vi "DUAL GAUGE-convert2int.vi"(0 "String in":string, 2 "W/R [W: Int in; Str out ]":bool, 9 "Integer1 in":u8, 11 "Integer2 in":u8) -> (4 "String out":string, 6 "Integer1 out":u8, 8 "Integer2 out":u8, 10 "Integer3 out":u8, 15 "Integer4 out":u8)   [LabVIEW 2010, in "Dual Gauge.lvlib"]
uses:
  Dual Gauge.lvlib
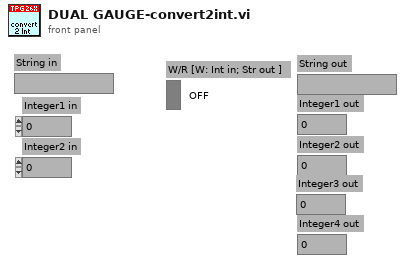
[diagram p1: front panel]
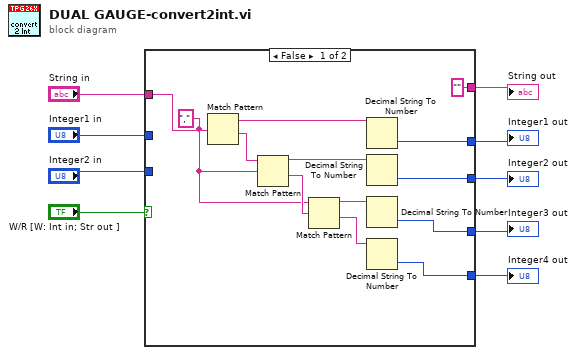
[diagram p0: block diagram]
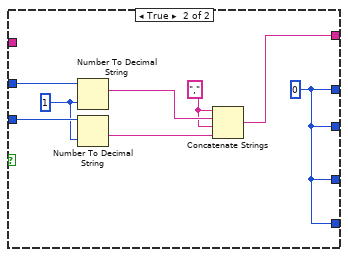
[diagram p2: hidden frame]
diagram:
  n1 = case shown="False" "W/R [W: Int in; Str out ]" {
    tunnel: "Integer1 in" -> [_ w30]
    tunnel: "Integer2 in" -> [_ w29]
    tunnel: ["" w28] -> w6
    tunnel: "String in" -> [w22 _]
    tunnel: [w20 w23] -> w4
    tunnel: [w19 w23] -> w3
    tunnel: [w12 w23] -> w2
    tunnel: [w11 w23] -> w1
    frame False {
      w10 = "," ("regular expression")
      n2 = Match Pattern(string=w22, regular expression=w10) -> (before substring=w21:string, after substring=w17:string)  [unwired: 1 in, 2 out]
      n3 = Match Pattern(string=w17, regular expression=w10) -> (before substring=w16:string, after substring=w15:string)  [unwired: 1 in, 2 out]
      n4 = Match Pattern(string=w10, regular expression=w15) -> (before substring=w14:string, after substring=w13:string)  [unwired: 1 in, 2 out]
      n5 = Decimal String To Number(string=w21) -> (number=w20:i32)  [unwired: 2 in, 1 out]
      n6 = Decimal String To Number(string=w16) -> (number=w19:i32)  [unwired: 2 in, 1 out]
      n7 = Decimal String To Number(string=w14) -> (number=w12:i32)  [unwired: 2 in, 1 out]
      n8 = Decimal String To Number(string=w13) -> (number=w11:i32)  [unwired: 2 in, 1 out]
    }
    frame True {
      w24 = ","
      w23 = 0
      w25 = i16 1 ("width (-)")
      n9 = Number To Decimal String(number=w30, width (-)=w25) -> (decimal integer string=w27:string)
      n10 = Number To Decimal String(number=w29, width (-)=w25) -> (decimal integer string=w26:string)
      n11 = Concatenate Strings(w24, w27, w24, w26) -> (w28:string)
    }
  }
  "Integer1 out" <- w4
  "Integer2 out" <- w3
  "String out" <- w6
  "Integer3 out" <- w2
  "Integer4 out" <- w1
